vi "Breakdown_list.vi"(8 "error in (no error)":errorcluster, 10 "Reason Type":T1, 11 "Ref In":T2={"MS SQL Connection"=refnum, "UDL File"=path "", "Time"="", "DCODE"="", "WIP+1"=0, "MC No?"=0, "POKAYOKE?"=FALSE, "Expected Result"="", "Result [Status]"="", "Clock"=0.0, "RFID"="", "WIP Queue"=refnum, "TS Parameter"={"ProfitCenterCode"="", "LineCode"="", "WorkOrderNumber"="", "Model"="", "Model_with_Prefix"="", "VendorCode"="", "SetParameterDateCode"="", "PokaYoke"=0, "Target"=1, "Live_DateCode"="", "CustomerPartNumber"="", "Hand"="", "sBarcode"=FALSE, "FCA"=0, "Ent_Stamp"=timestamp(0 s since 1904-01-01), "STS_CD"=0.0}, "Data_Queue"=[], "RFID Serial No."=""} {"TS Parameter"."FCA" format="%01d"; "TS Parameter"."Target" min=1 max=100000; "TS Parameter"."PokaYoke" min=0 max=1}) -> (0 "error out":errorcluster, 1 "Data":string[][](array[string]), 2 "Reason List":string[](array[string]), 3 "List":string[](array[string]))   [LabVIEW 2020]
uses:
  Controls/TD SQL.ctl
  <vilib>/addons/database/Connection.llb/Conn ObjectReference.ctl
  Controls/WIP_State.ctl
  Controls/TS_Parameter.ctl
  Controls/Loss_type.ctl
  <vilib>/addons/database/_DB Variant To Data/Database Variant To Data.xnode
  <vilib>/addons/database/NI_Database_API.lvlib
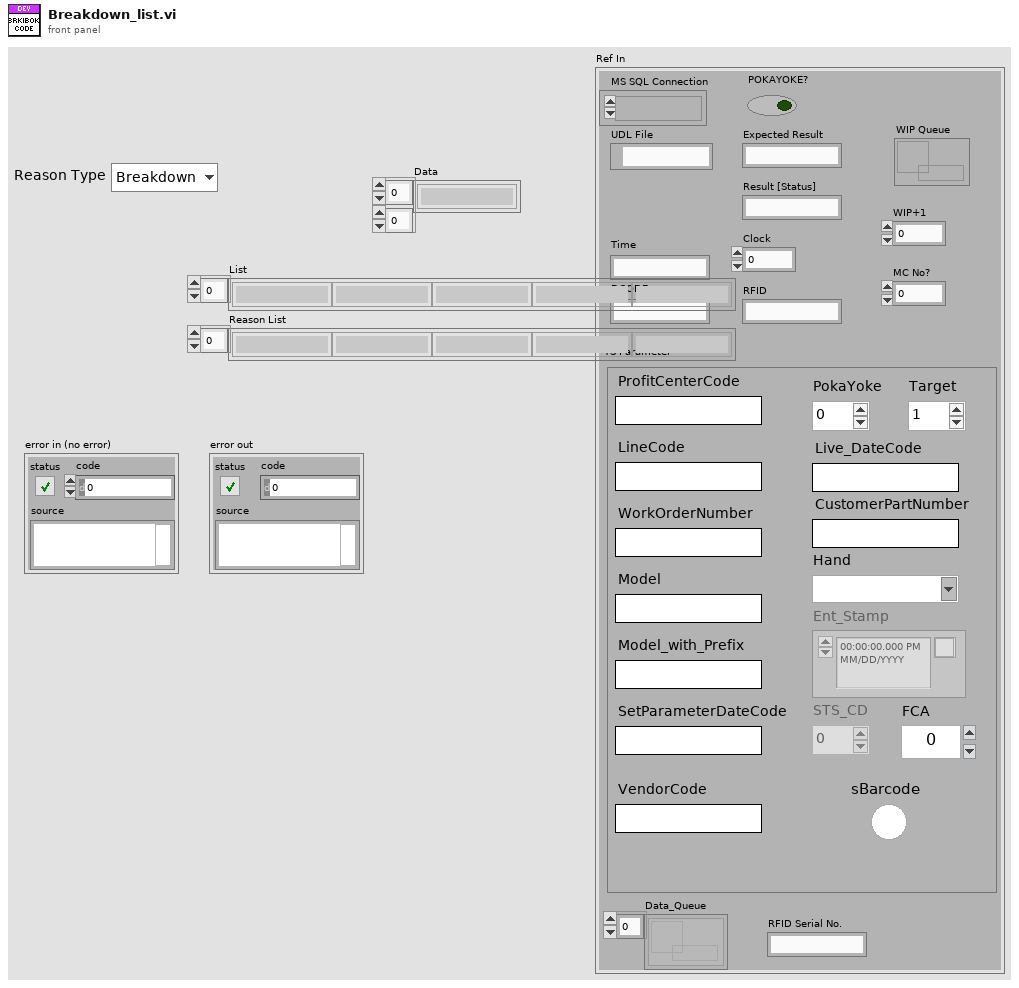
[diagram p1: front panel]
types:
  T1 = typedef "Loss_type.ctl" = enum16{"Breakdown", "Bookout"}
  T2 = typedef "TD SQL.ctl" = cluster{"MS SQL Connection":T3, "UDL File":path, "Time":string, "DCODE":string, "WIP+1":i64, "MC No?":i32, "POKAYOKE?":bool, "Expected Result":string, "Result [Status]":string, "Clock":dbl, "RFID":string, "WIP Queue":refnum<queue>, "TS Parameter":T4, "Data_Queue":refnum<queue>[], "RFID Serial No.":string}
  T3 = typedef "NI_Database_API.lvlib/Conn ObjectReference.ctl" = refnum<k1>
  T4 = typedef "TS_Parameter.ctl" = cluster{"ProfitCenterCode":string, "LineCode":string, "WorkOrderNumber":string, "Model":string, "Model_with_Prefix":string, "VendorCode":string, "SetParameterDateCode":string, "PokaYoke":i32, "Target":i32, "Live_DateCode":string, "CustomerPartNumber":string, "Hand":string, "sBarcode":bool, "FCA":i32, "Ent_Stamp":timestamp, "STS_CD":dbl}
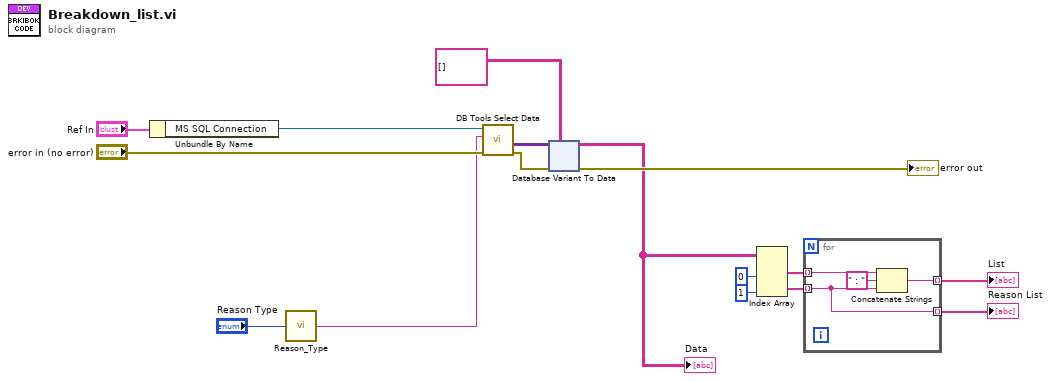
[diagram p0: block diagram]
diagram:
  n1 = Unbundle By Name("Ref In") -> ("MS SQL Connection"=w15:T3)
  n2 = call "Reason_Type.vi"("Reason Type"="Reason Type") -> ("Break|Bookout"=w4:string)  [unwired: 2 in, 1 out]
  n3 = call <vilib>:"DB Tools Select Data.vi"("error in (no error)"="error in (no error)", "table"=w4, "connection reference"=w15) -> ("error out"=w12:errorcluster, "data"=w10:variant[][])  [unwired: 3 in, 1 out]
  n4 = xnode "Database Variant To Data"("database variant"=w10, "error in (no error)"=w12, "type"=string[][] []) -> ("data"=w5:string[][], "error out"=→"error out":errorcluster)
  "Data" <- w5
  n5 = Index Array(array=w5, index (col) #1=0 ("disabled index (col)"), index (col) #2=1 ("index (col)")) -> (element #1=w7:string[], element #2=w6:string[])  [unwired: 2 in]
  n6 = for {
    tunnel: w7 -> [w20] mode=indexing
    tunnel: w6 -> [w17] mode=indexing
    tunnel: [w18] -> w2 mode=indexing
    tunnel: [w17] -> w1 mode=indexing
    n7 = Concatenate Strings(w20, " : " ("string"), w17) -> (w18:string)
  }
  "List" <- w2
  "Reason List" <- w1
